vi "Save Copy of Class.vi"(8 "error in (no error)":errorcluster, 11 "QControl Creation in":refnum<class "QControl Creation.lvclass">) -> (0 "error out":errorcluster, 3 "QControl Creation out":refnum<class "QControl Creation.lvclass">)   [LabVIEW 2015, in "QControl Creation.lvclass"]
doc: "<b> </b> <b> </b>\n©2016 Q Software Innovations, LLC (QSI)\nwritten by Quentin Alldredge\nproduced in LabVIEW 2015\n\nsupport@qsoftwareinnovations.com\nwww.qsoftwareinnovations.com\n\nAll rights reserved.\n\nRedistribution and use in source and binary forms, with or without modification, are permitted provided that the following conditions are met:\n\n * Redistributions of source code must retain the above copyright notice, this list of conditions and the following disclaimer.\n * Redistributions in binary form must reproduce the above copyright notice, this list of conditions and the following disclaimer in the documentation and/or other materials provided with the distribution.\n * Neither the name of Q Software Innovations, LLC. nor the names of its contributors may be used to endorse or promote products derived from this software without specific prior written permission.\n\nTHIS SOFTWARE IS PROVIDED BY THE COPYRIGHT HOLDERS AND CONTRIBUTORS \"AS IS\" AND ANY EXPRESS OR IMPLIED WARRANTIES, INCLUDING, BUT NOT LIMITED TO, THE IMPLIED WARRANTIES OF MERCHANTABILITY AND FITNESS FOR A PARTICULAR PURPOSE ARE DISCLAIMED. IN NO EVENT SHALL THE COPYRIGHT OWNER OR CONTRIBUTORS BE LIABLE FOR ANY DIRECT, INDIRECT, INCIDENTAL, SPECIAL, EXEMPLARY, OR CONSEQUENTIAL DAMAGES (INCLUDING, BUT NOT LIMITED TO, PROCUREMENT OF SUBSTITUTE GOODS OR SERVICES; LOSS OF USE, DATA, OR PROFITS; OR BUSINESS INTERRUPTION) HOWEVER CAUSED AND ON ANY THEORY OF LIABILITY, WHETHER IN CONTRACT, STRICT LIABILITY, OR TORT (INCLUDING NEGLIGENCE OR OTHERWISE) ARISING IN ANY WAY OUT OF THE USE OF THIS SOFTWARE, EVEN IF ADVISED OF THE POSSIBILITY OF SUCH DAMAGE."
uses:
  QControl Creation.lvclass
  QControl Creation.lvclass/QControl Creation.ctl
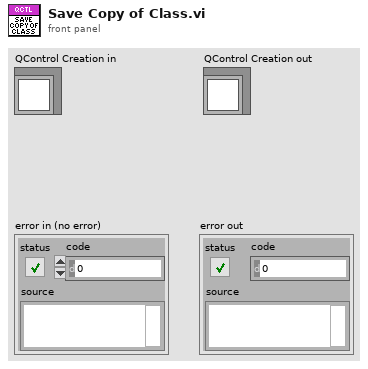
[diagram p1: front panel]
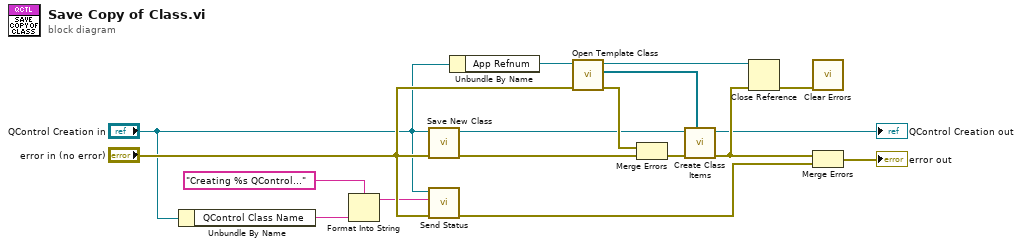
[diagram p0: block diagram]
diagram:
  n1 = Unbundle By Name("QControl Creation in") -> ("QControl Class Name"=w2:string)
  n2 = Format Into String(format string="Creating %s QControl..." ("Value"), w2) -> (resulting string=w1:string)  [unwired: 2 in, 1 out]
  n3 = call "Save New Class.vi"("error in (no error)"="error in (no error)", "QControl Creation in"="QControl Creation in") -> ("error out"=w10:errorcluster, "QControl Creation out"=w6:refnum<class "QControl Creation.lvclass">)  [unwired: 7 in, 1 out]
  n4 = call "Send Status.vi"("error in (no error)"="error in (no error)", "Status"=w1, "QControl Creation in"="QControl Creation in") -> ("error out (dup)"=w8:errorcluster)  [unwired: 7 in, 1 out]
  n5 = Unbundle By Name("QControl Creation in") -> ("App Refnum"=w13:refnum<vi>)
  n6 = call "Open Template Class.vi"("error in (no error)"="error in (no error)", "Application in"=w13) -> ("error out"=w14:errorcluster, "Template Class Methods and Controls"=w7:refnum<vi>[], "Template Class Refnum out"=w15:refnum<vi>)  [unwired: 7 in]
  n7 = Merge Errors(w14, w10) -> (w11:errorcluster)
  n8 = call "Create Class Items.vi"("Template Class Items"=w7, "error in (no error)"=w11, "QControl Creation in"=w6) -> ("error out"=w17:errorcluster, "QControl Creation out"=→"QControl Creation out":refnum<class "QControl Creation.lvclass">)  [unwired: 7 in]
  n9 = Close Reference(reference=w15, error in (no error)=w17) -> (error out=w16:errorcluster)
  n10 = call <vilib>:"Clear Errors.vi"("error in (no error)"=w16) -> ()  [unwired: 5 in, 2 out]
  n11 = Merge Errors(w17, w8) -> (→"error out":errorcluster)
